vi "Validate Fixed Header.vi"(8 "error in (no error)":errorcluster, 11 "PUBACK in":refnum<class "PUBACK.lvclass">) -> (0 "error out":errorcluster, 1 "Valid":bool, 3 "PUBACK out":refnum<class "PUBACK.lvclass">)   [LabVIEW 2013, in "PUBACK.lvclass"]
uses:
  PUBACK.lvclass
  ControlPacket/ControlPacket.lvclass/ControlPacket.ctl
  ControlPacket/ControlPacket.lvclass
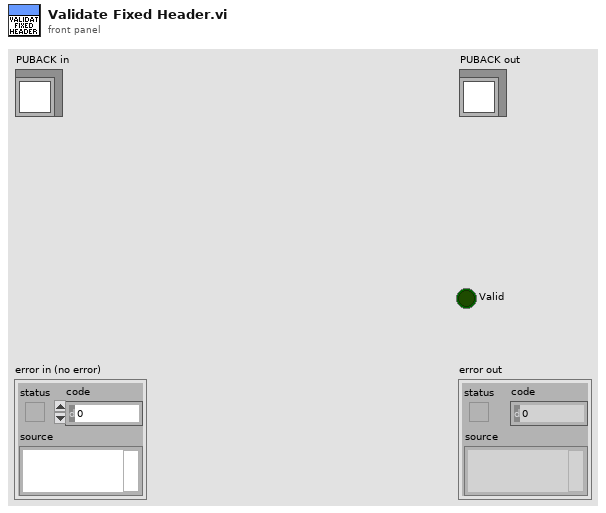
[diagram p1: front panel]
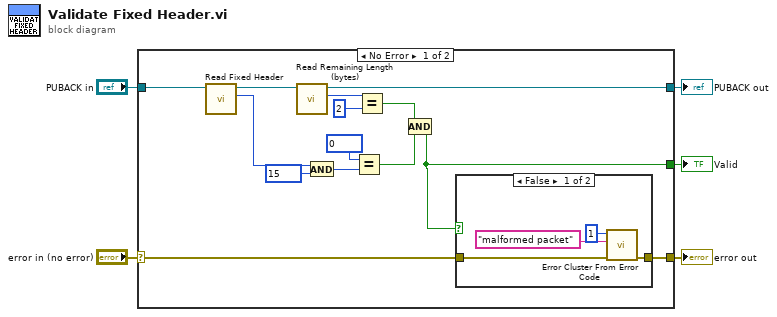
[diagram p0: block diagram]
diagram:
  n1 = case shown="No Error" "error in (no error)" {
    selector: "error in (no error)" -> [w17 w26]
    tunnel: [w16 w26] -> w3
    tunnel: [w6 _] -> w2
    tunnel: [w11 w25] -> w1
    tunnel: "PUBACK in" -> [w18 w25]
    frame No Error {
      n2 = call "Read Fixed Header.vi"("ControlPacket in"=w18) -> ("Fixed Header"=w15:u8, "ControlPacket out"=w12:refnum<class "PUBACK.lvclass">)  [unwired: 9 in]
      n3 = call "Read Remaining Length (bytes).vi"("ControlPacket in"=w12) -> ("Remaining Length (bytes)"=w10:u32, "ControlPacket out"=w11:refnum<class "PUBACK.lvclass">)  [unwired: 8 in, 1 out]
      n4 = And(x=w15, y=u8 15) -> (x .and. y?=w14:u8)
      n5 = Equal?(x=u8 0 ("y"), y=w14) -> (x = y?=w7:bool)
      n6 = Equal?(x=w10, y=u32 2) -> (x = y?=w8:bool)
      n7 = Compound Arithmetic op=AND(w8, w7) -> (w6:bool)
      n8 = case shown="False" w6 {
        tunnel: [w21 w24] -> w16
        tunnel: w17 -> [w20 w24]
        frame False {
          n9 = call <vilib>:"Error Cluster From Error Code.vi"("error in (no error)"=w20, "error message (\"\")"="malformed packet" ("error message (\"\")"), "error code (0)"=1) -> ("error out"=w21:errorcluster)  [unwired: 6 in]
        }
        frame True {
        }
      }
    }
    frame Error {
    }
  }
  "Valid" <- w2
  "error out" <- w3
  "PUBACK out" <- w1
